vi "Begin.vi"(8 "error in (no error)":errorcluster, 10 "variant in":variant, 11 "Panzer in":refnum<class "Panzer.lvclass">) -> (0 "error out":errorcluster, 3 "Panzer out":refnum<class "Panzer.lvclass">)   [LabVIEW 2019, in "Robot.lvlib" / "Panzer.lvclass"]
uses:
  Panzer.lvclass
  Robot.lvclass
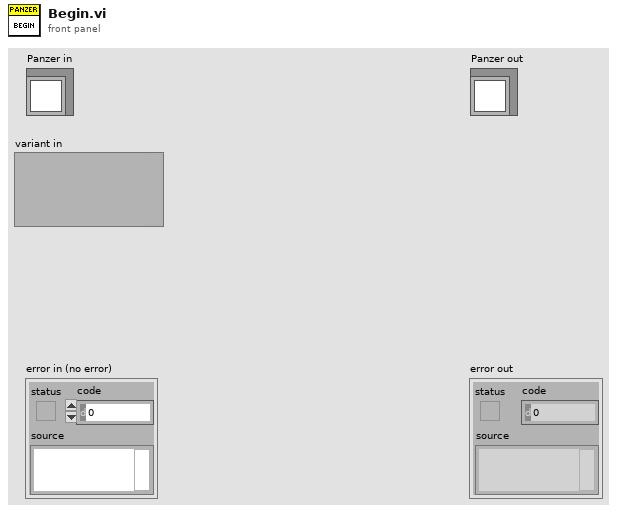
[diagram p1: front panel]
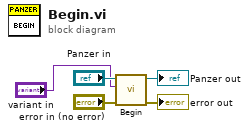
[diagram p0: block diagram]
diagram:
  n1 = call-parent "Begin.vi"("error in (no error)"="error in (no error)", "variant in"="variant in", "Robot in"="Panzer in") -> ("error out"=→"error out":errorcluster, "Robot out"=→"Panzer out":refnum<class "Panzer.lvclass">)  [unwired: 7 in]
